vi "Get Pin Name.vi"(8 "error in (no error)":errorcluster, 11 "pin map":path) -> (0 "error out":errorcluster, 3 "Pin Name":string[](array[string]))   [LabVIEW 2018]
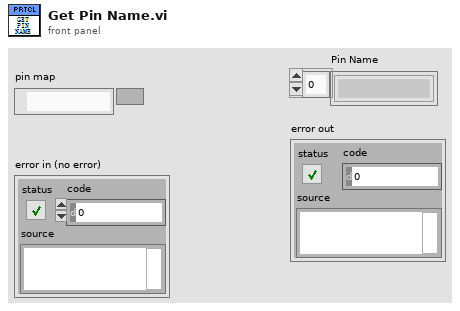
[diagram p1: front panel]
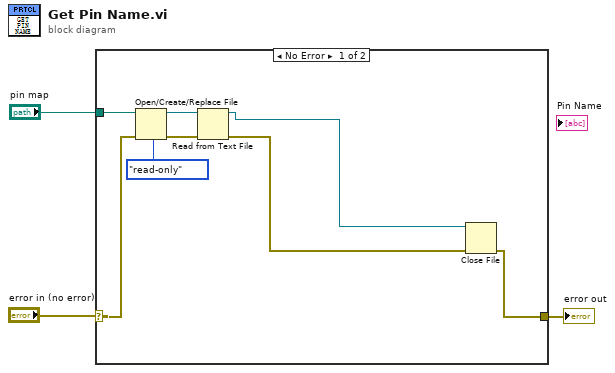
[diagram p0: block diagram]
diagram:
  n1 = case shown="No Error" "error in (no error)" {
    selector: "error in (no error)" -> [w7 w12]
    tunnel: [w8 w12] -> w2
    tunnel: "pin map" -> [w11 _]
    frame No Error {
      n2 = Open/Create/Replace File(file path (use dialog)=w11, error in=w7, access (0:read/write)=enum16{"read/write", "read-only", "write-only"}."read-only") -> (refnum out=w10:refnum<file>, error out=w9:errorcluster)  [unwired: 3 in, 1 out]
      n3 = Read from Text File(file (use dialog)=w10, error in=w9) -> (refnum out=w5:refnum<file>, error out=w4:errorcluster)  [unwired: 2 in, 2 out]
      n4 = Close File(refnum=w5, error in=w4) -> (error out=w8:errorcluster)  [unwired: 1 out]
    }
    frame Error {
    }
  }
  "error out" <- w2
